vi "Flatten.vi"(8 "error in (no error)":errorcluster, 11 "Voltage Pulse Gating System (HV supply) in":refnum<class "Voltage Pulse Gating System (HV supply).lvclass">) -> (0 "error out":errorcluster, 3 "Voltage Pulse Gating System (HV supply) out":refnum<class "Voltage Pulse Gating System (HV supply).lvclass">)   [LabVIEW 2017, in "Voltage Pulse Gating System (HV supply).lvclass"]
uses:
  Voltage Pulse Gating System (HV supply).lvclass
  Global/File Locations.vi
  Scanner/Scanner.lvclass
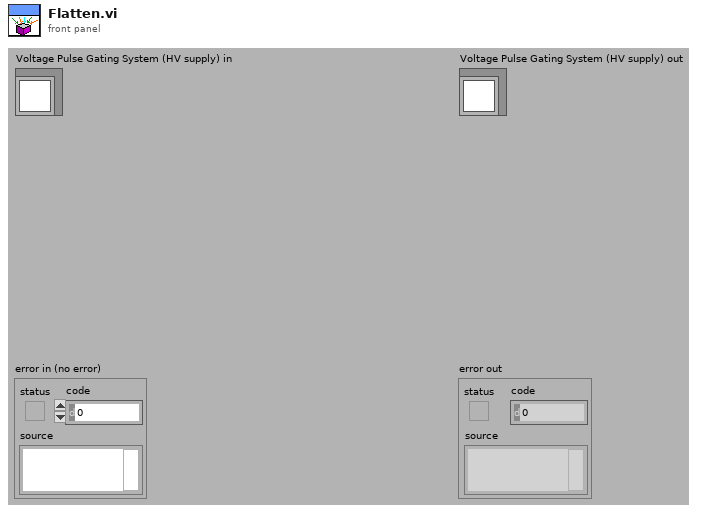
[diagram p1: front panel]
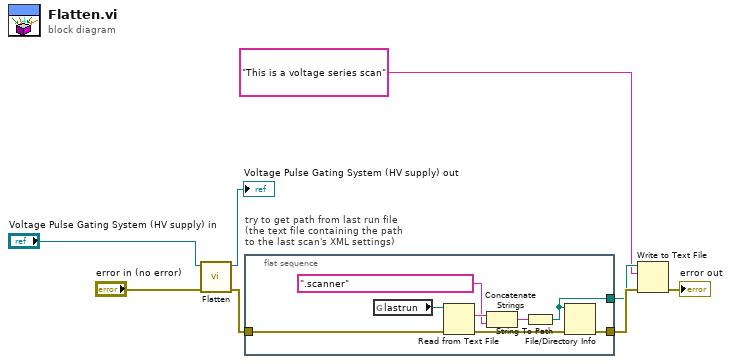
[diagram p0: block diagram]
diagram:
  n1 = call-parent "Flatten.vi"("error in (no error)"="error in (no error)", "Scanner in"="Voltage Pulse Gating System (HV supply) in") -> ("error out"=w8:errorcluster, "Scanner out"=→"Voltage Pulse Gating System (HV supply) out":refnum<class "Voltage Pulse Gating System (HV supply).lvclass">)  [unwired: 8 in]
  n2 = flat-sequence "try to get path from last run file\n(the text file containing the path\nto the last scan's XML settings)" {
    tunnel: [w16] -> w6
    tunnel: [w13] -> w7
    tunnel: w8 -> [w12]
    frame #0 {
      n3 = global read "File Locations.vi" "lastrun"() -> (w15:path)
      n4 = Read from Text File(file (use dialog)=w15, error in=w12) -> (text=w11:string, error out=w14:errorcluster)  [unwired: 4 out]
      n5 = Concatenate Strings(w11, ".scanner") -> (w9:string)
      n6 = String To Path(string=w9) -> (path=w16:path)
      n7 = File/Directory Info(path=w16, error in=w14) -> (error out=w13:errorcluster)  [unwired: 6 out]
    }
  }
  n8 = Write to Text File(file (use dialog)=w6, text="This is a voltage series scan" ("format string"), error in=w7) -> (error out=→"error out":errorcluster)  [unwired: 1 in, 2 out]
